vi "TestDeviceLoading.vi"() -> ()   [LabVIEW 2018]
panel:
  in  "MG17Motor 3":refnum<k7>(container)
  in  "MG17Motor 2":refnum<k7>(container)
  in  "MG17Motor":refnum<k7>(container)
  in  "MG17System":refnum<k7>(container)
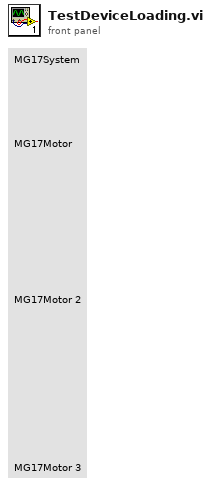
[diagram p1: front panel]
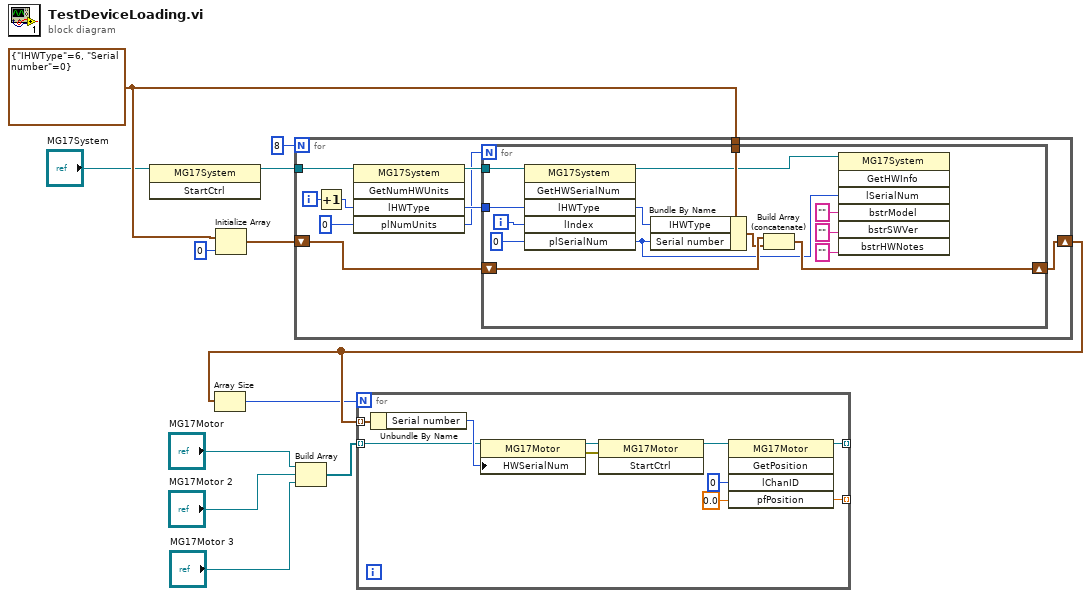
[diagram p0: block diagram]
diagram:
  w10 = cluster{"IHWType":i32, "Serial number":i32} {"IHWType"=6, "Serial number"=0}
  n1 = invoke class="MG17System" method="StartCtrl"(reference="MG17System") -> (reference out=w12:refnum<k7>)  [unwired: 2 in, 2 out]
  n2 = Initialize Array(w10, 0 ("dimension size")) -> (w8:cluster{"IHWType":i32, "Serial number":i32}[])
  n3 = for {
    N: 8 -> [_]
    tunnel: w12 -> [w22]
    shift-right: [w13] -> w7
    shift-left: w8 -> [w14]
    tunnel: w10 -> [w15]
    i -> [w17]
    n4 = Increment(x=w17) -> (x+1=w16:i32)
    n5 = invoke class="MG17System" method="GetNumHWUnits"(reference=w22, "lHWType"=w16, "plNumUnits"=0) -> (reference out=w20:refnum<k7>, "lHWType"=w19:i32, "plNumUnits"=w18:i32)  [unwired: 2 in, 2 out]
    n6 = for {
      N: w18 -> [_]
      tunnel: w20 -> [w36]
      tunnel: w19 -> [w35]
      tunnel: w15 -> [w32]
      shift-right: [w29] -> w13
      shift-left: w14 -> [w30]
      i -> [w33]
      n7 = invoke class="MG17System" method="GetHWSerialNum"(reference=w36, "lHWType"=w35, "lIndex"=w33, "plSerialNum"=0) -> (reference out=w27:refnum<k7>, "lHWType"=w31:i32, "plSerialNum"=w26:i32)  [unwired: 2 in, 3 out]
      n8 = Bundle By Name(cluster=w32, "IHWType"=w31, "Serial number"=w26) -> (w28:cluster{"IHWType":i32, "Serial number":i32})
      n9 = Build Array (concatenate)(w30, w28) -> (w29:cluster{"IHWType":i32, "Serial number":i32}[])
      n10 = invoke class="MG17System" method="GetHWInfo"(reference=w27, "lSerialNum"=w26, "bstrModel"="", "bstrSWVer"="", "bstrHWNotes"="") -> ()  [unwired: 2 in, 7 out]
    }
  }
  n11 = Array Size(array=w7) -> (size(s)=w5:i32)
  n12 = Build Array("MG17Motor", "MG17Motor 2", "MG17Motor 3") -> (w1:refnum<k7>[])
  n13 = for {
    N: w5 -> [_]
    tunnel: w7 -> [w46] mode=indexing
    tunnel: w1 -> [w38] mode=indexing
    tunnel: [w39] -> _ mode=indexing
    tunnel: [w37] -> _ mode=indexing
    n14 = Unbundle By Name(w46) -> ("Serial number"=w45:i32)
    n15 = property class="MG17Motor"(reference=w38, "HWSerialNum"=w45) -> (reference out=w44:refnum<k7>, error out=w43:errorcluster)  [unwired: 1 in]
    n16 = invoke class="MG17Motor" method="StartCtrl"(reference=w44, error in=w43) -> (reference out=w42:refnum<k7>)  [unwired: 1 in, 2 out]
    n17 = invoke class="MG17Motor" method="GetPosition"(reference=w42, "lChanID"=0, "pfPosition"=sgl 0.0) -> (reference out=w37:refnum<k7>, "pfPosition"=w39:sgl)  [unwired: 2 in, 3 out]
  }
